vi "tm_getelectroninfo_40.vi"(8 "error in (no error)":errorcluster, 11 "Handle in":u32) -> (0 "error out":errorcluster, 1 "Coefficient":sgl, 2 "Offset":sgl, 3 "Handle out":u32)   [LabVIEW 2023]
uses:
  tmcamcon.dll
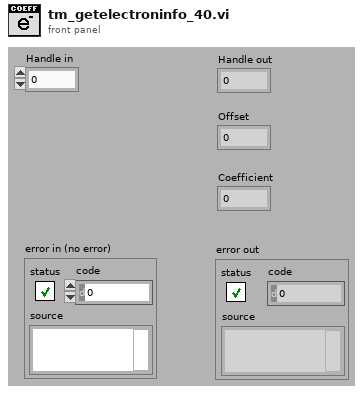
[diagram p1: front panel]
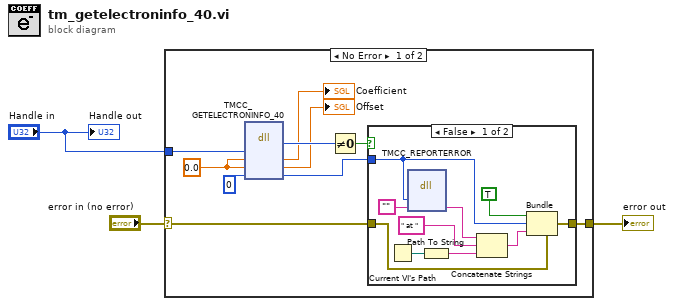
[diagram p0: block diagram]
diagram:
  n1 = case shown="No Error" "error in (no error)" {
    selector: "error in (no error)" -> [w12 w25]
    tunnel: [w11 w25] -> w2
    tunnel: "Handle in" -> [w4 _]
    frame No Error {
      w7 = sgl 0.0 ("coeff")
      n2 = dll-call lib="tmcamcon.dll" fn="TMCC_GETELECTRONINFO_40"("handle"=w4, "coeff"=w7, "offset"=w7, "Erval"=0) -> ("return type"=w8:u32, "coeff"=→"Coefficient":sgl, "offset"=→"Offset":sgl, "Erval"=w9:i32)  [unwired: 4 in, 2 out]
      n3 = Not Equal To 0?(x=w8) -> (x != 0?=w13:bool)
      n4 = case shown="False" w13 {
        tunnel: w12 -> [w23 w24]
        tunnel: [w22 w24] -> w11
        tunnel: w9 -> [w16 _]
        frame False {
          n5 = Current VI's Path() -> (path=w21:path)
          n6 = dll-call lib="tmcamcon.dll" fn="TMCC_REPORTERROR"("error"=w16, "buf"="") -> ("buf"=w15:string)  [unwired: 5 in, 2 out]
          n7 = Path To String(path=w21) -> (string=w17:string)
          n8 = Concatenate Strings(w15, " at ", w17) -> (w20:string)
          n9 = Bundle(cluster=w23, "status"=TRUE, "code"=w16, "source"=w20) -> (w22:errorcluster)
        }
        frame True {
        }
      }
    }
    frame Error {
    }
  }
  "error out" <- w2
  "Handle out" <- "Handle in"
